vi "Untitled 1.vi"() -> ()   [LabVIEW 2011]
uses:
  System.Drawing
panel:
  out "stripped path":path
  out "error out":errorcluster
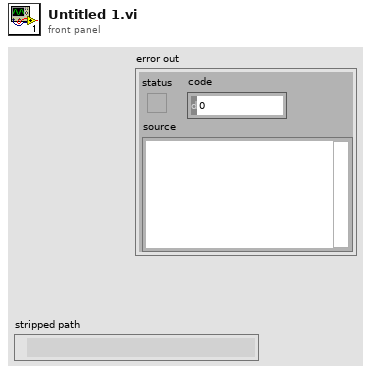
[diagram p1: front panel]
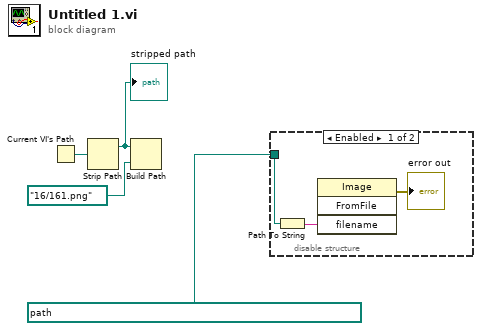
[diagram p0: block diagram]
diagram:
  n1 = Current VI's Path() -> (path=w4:path)
  n2 = Strip Path(path=w4) -> (stripped path=w3:path)  [unwired: 1 out]
  "stripped path" <- w3
  n3 = Build Path(base path=w3, name or relative path=path "16/161.png" ("路径")) -> ()  [unwired: 1 out]
  n4 = disable-structure shown="Enabled" {
    disable-tunnel: path "E:/BOOK/功能块/NET工具/NET控件/ListView/32/324.png" ("appended path") -> [w5 _]
    frame Enabled {
      n5 = Path To String(path=w5) -> (string=w7:string)
      n6 = invoke class="Image" method="FromFile"("filename"=w7) -> (error out=→"error out":errorcluster)  [unwired: 3 in, 3 out]
    }
    frame Disabled {
    }
  }
